vi "storeADCMixedToArray-wang-test2simplifié.vi"(0 "String":string) -> (18 "Graph Data":T1)   [LabVIEW 2014]
uses:
  main/controls/Graph Data.ctl
  <vilib>/Utility/miscctls.llb/LVAnnotationListTypeDef.ctl
  <vilib>/Utility/miscctls.llb/LVCursorListTypeDef.ctl
panel:
  out "Numeric 3":i32
  out "TotalTrigger 2":i32
  out "Array - Numeric":i32[](array[numeric])
  out "counter":i32
  in  "counterc":i32
  out "header string":string
  out "channel":u8[](array[numeric])
  out "Waveform":waveform(dbl)
  out "Graph":waveform(i32)[](graph)
  out "Numeric 2":i32
  out "Numeric":i32
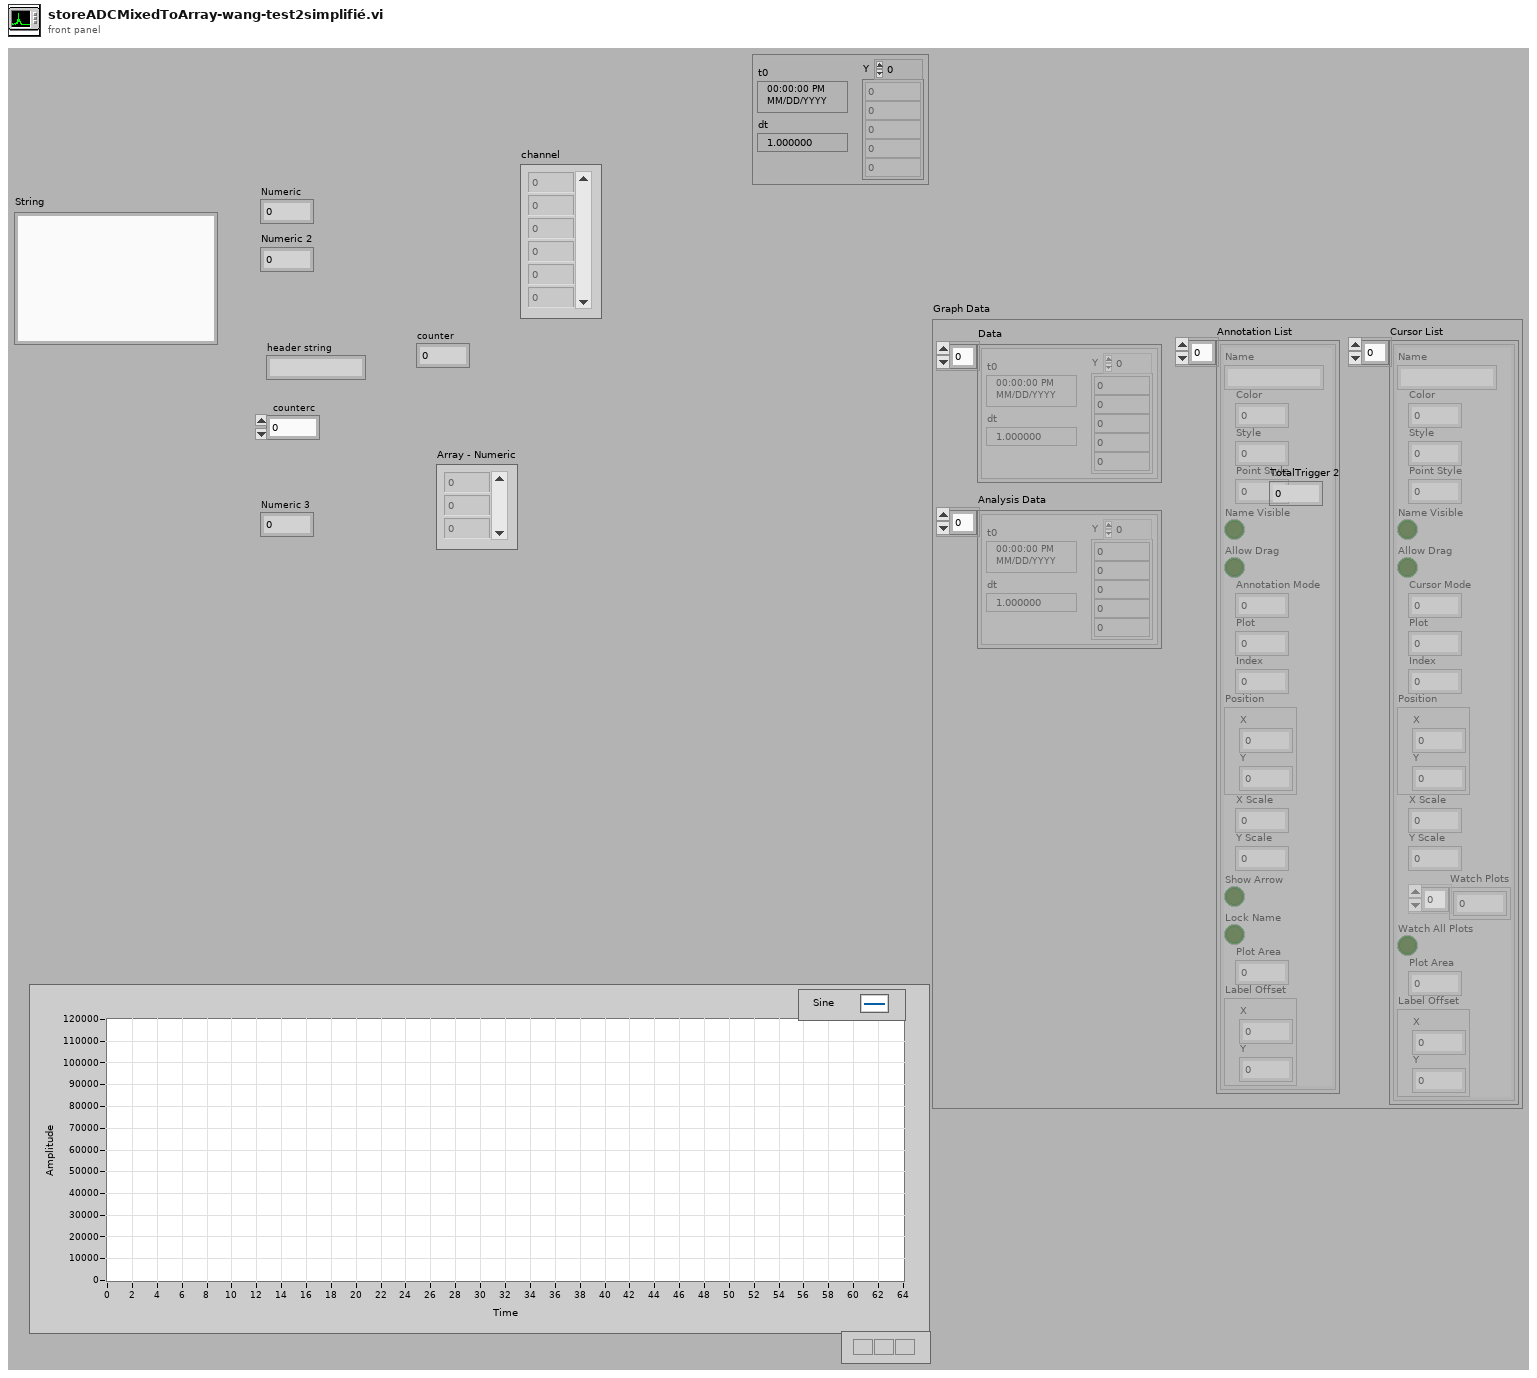
[diagram p1: front panel]
types:
  T1 = typedef "Graph Data.ctl" = cluster{"Data":waveform(dbl)[], "Annotation List":T2, "Cursor List":T3, "Analysis Data":waveform(dbl)[]}
  T2 = typedef "LVAnnotationListTypeDef.ctl" = cluster{"Name":string, "Color":u32, "Style":u8, "Point Style":u8, "Name Visible":bool, "Allow Drag":bool, "Annotation Mode":u32, "Plot":i32, "Index":i32, "Position":cluster{"X":dbl, "Y":dbl}, "X Scale":u32, "Y Scale":u32, "Show Arrow":bool, "Lock Name":bool, "Plot Area":i32, "Label Offset":cluster{"X":dbl, "Y":dbl}}[]
  T3 = typedef "LVCursorListTypeDef.ctl" = cluster{"Name":string, "Color":u32, "Style":u8, "Point Style":u8, "Name Visible":bool, "Allow Drag":bool, "Cursor Mode":u32, "Plot":i32, "Index":i32, "Position":cluster{"X":dbl, "Y":dbl}, "X Scale":u32, "Y Scale":u32, "Watch Plots":i32[], "Watch All Plots":bool, "Plot Area":i32, "Label Offset":cluster{"X":dbl, "Y":dbl}}[]
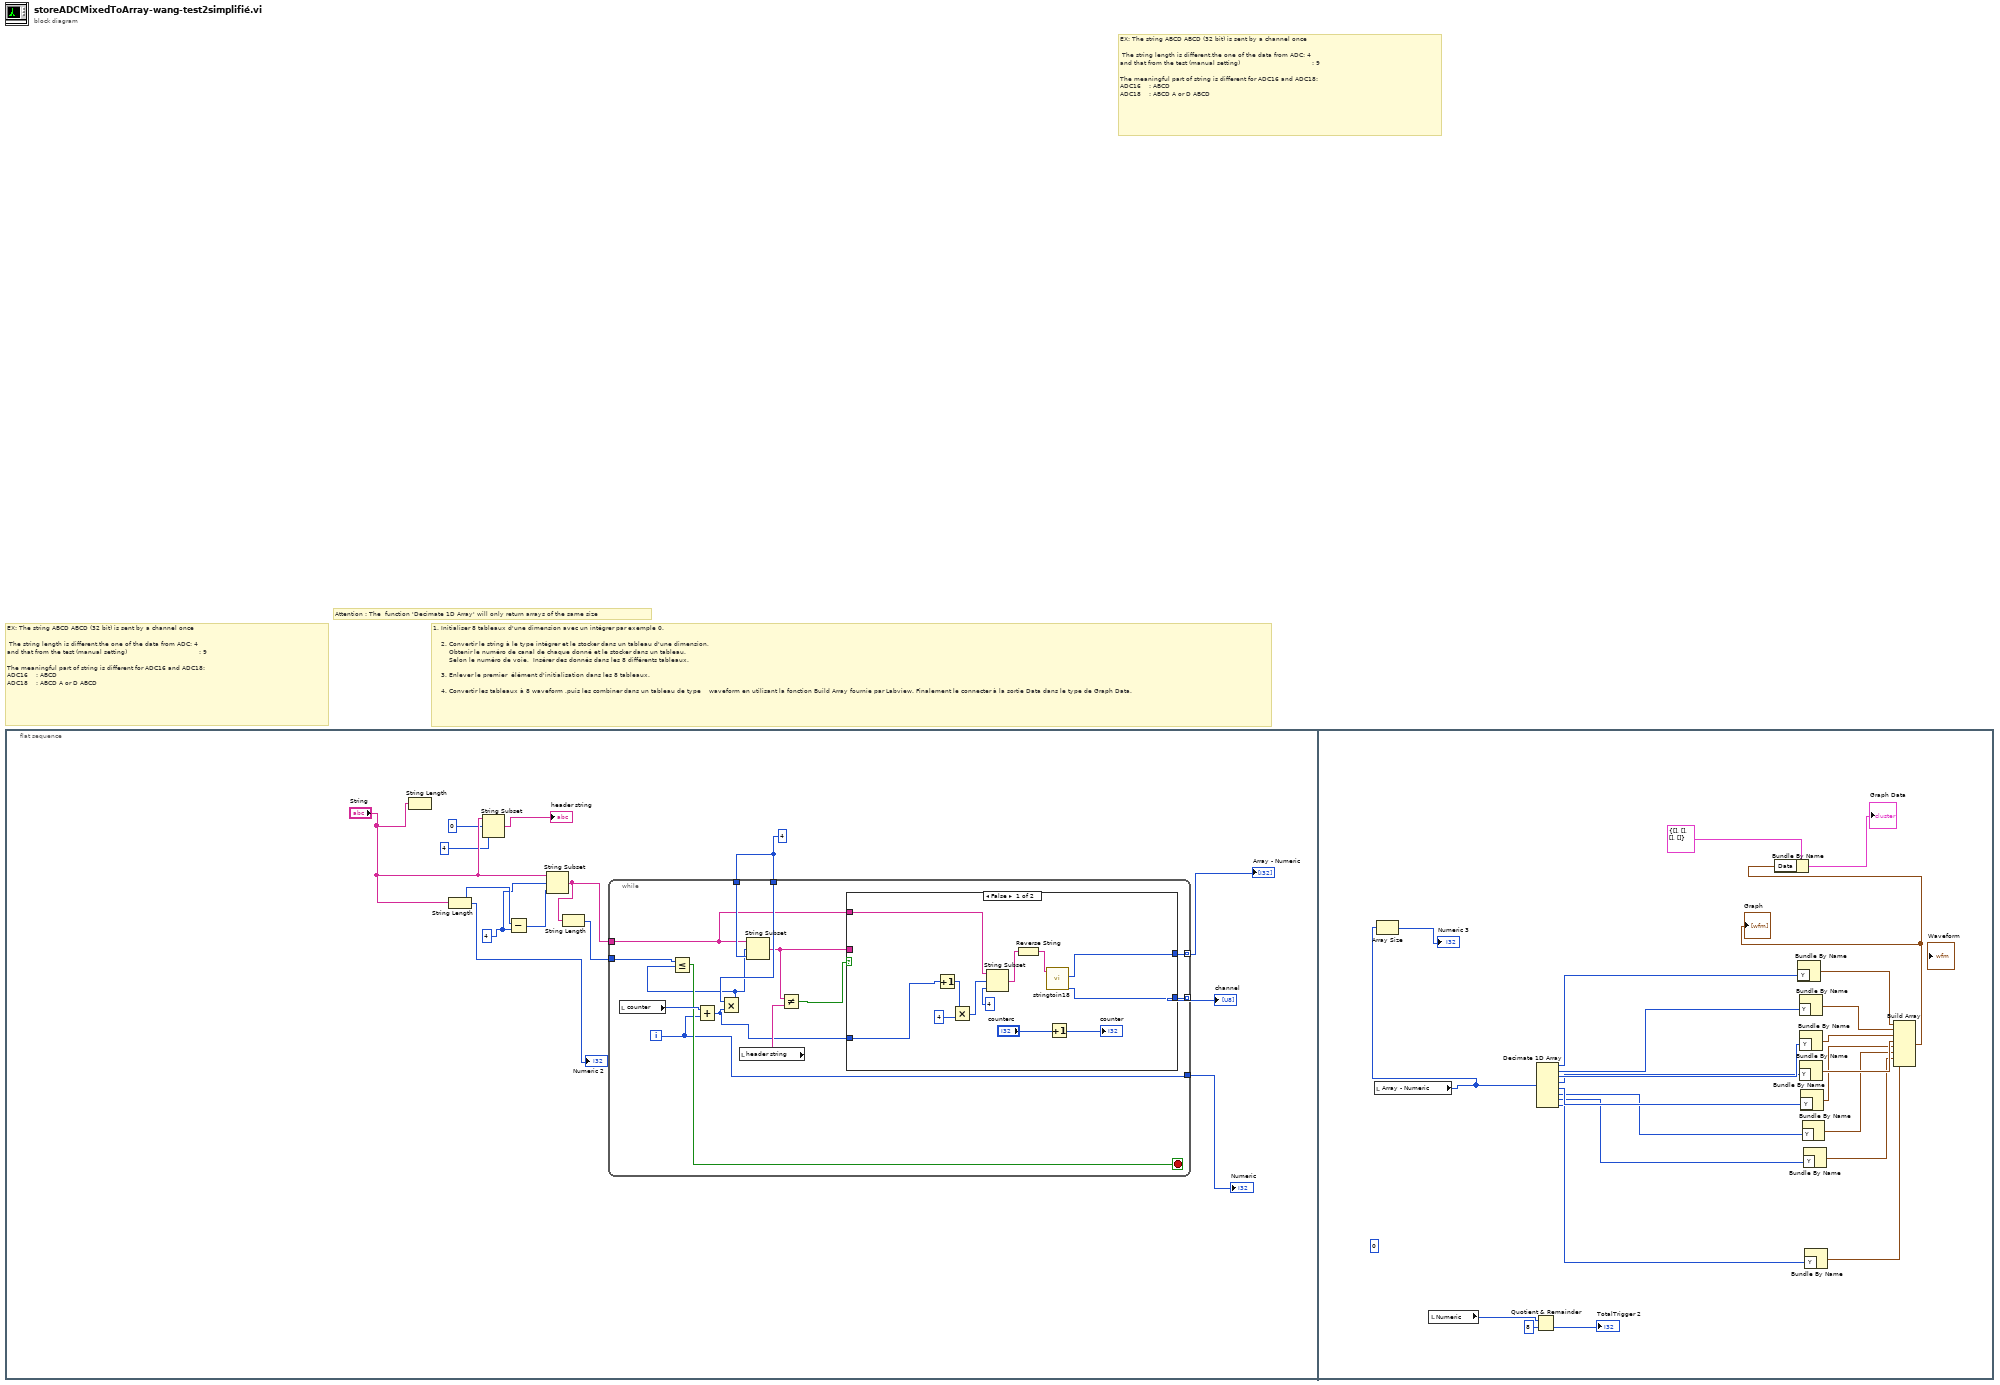
[diagram p0: block diagram]
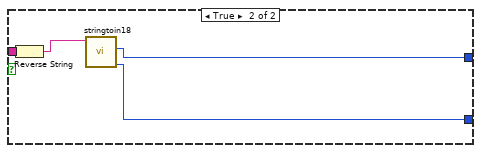
[diagram p2: hidden frame]
diagram:
  # "Attention : The  function 'Decimate 1D Array' will only return arrays of the same size"
  # "1. Initialiser 8 tableaux d'une dimension avec un intégrer par exemple 0.\n\n    2.\tConvertir le string à le type intégrer et le stocker dans un tableau d'une dimension,\n        Obtenir le numéro de canal de chaque donné et le stocker dans un tableau.  \n        Selon le numéro de voie,  Insérer des donnés dans les 8 différents tableaux.\n\n    3. Enlever le premier  élément d'initialisation dans les 8 tableaux.\n\n    4. Convertir les tableaux à 8 waveform ,puis les combiner dans un tableau de type    waveform en utilisant la fonction Build Array fournie par Labview. Finalement le connecter à la sortie Data dans le type de Graph Data."
  # "EX: The string ABCD ABCD (32 bit) is sent by a channel once                \n\n The string length is different,the one of the data from ADC: 4\nand that from the test (manual setting)                                    : 9\n\nThe meaningful part of string is different for ADC16 and ADC18:\nADC16    : ABCD                          \nADC18    : ABCD A or D ABCD"
  # "EX: The string ABCD ABCD (32 bit) is sent by a channel once                \n\n The string length is different,the one of the data from ADC: 4\nand that from the test (manual setting)                                    : 9\n\nThe meaningful part of string is different for ADC16 and ADC18:\nADC16    : ABCD                          \nADC18    : ABCD A or D ABCD"
  n1 = flat-sequence {
    frame #0 {
      w2 = 4
      w5 = 4
      n2 = String Length(string="String") -> ()  [unwired: 1 out]
      n3 = String Length(string="String") -> (length=w13:i32)
      "Numeric 2" <- w13
      n4 = String Subset(string="String", offset (0)=0, length (rest)=4 ("length (rest)")) -> (substring=→"header string":string)
      n5 = Subtract(x=w13, y=w5) -> (x-y=w11:i32)
      n6 = String Subset(string="String", offset (0)=w5, length (rest)=w11) -> (substring=w4:string)
      n7 = String Length(string=w4) -> (length=w3:i32)
      n8 = while {
        tunnel: w2 -> [w27]
        tunnel: w2 -> [w26]
        tunnel: [w16] -> w12
        tunnel: w4 -> [w21]
        tunnel: [w25] -> w1 mode=indexing
        tunnel: [w24] -> w10 mode=indexing
        tunnel: w3 -> [w18]
        i -> [w16]
        stop <- w17 stop-if-true
        n9 = local read "counter"() -> (w22:i32)
        n10 = Add(x=w22, y=w16) -> (x+y=w14:i32)
        n11 = Multiply(x=w26, y=w14) -> (x*y=w15:i32)
        n12 = Less Or Equal?(x=w18, y=w15) -> (x <= y?=w17:bool)
        n13 = local read "header string"() -> (w23:string)
        n14 = String Subset(string=w21, offset (0)=w15, length (rest)=w27) -> (substring=w20:string)
        n15 = Not Equal?(x=w20, y=w23) -> (x != y?=w19:bool)
        n16 = case shown="False" w19 {
          tunnel: [w35 w43] -> w25
          tunnel: [w34 w42] -> w24
          tunnel: w20 -> [_ w40]
          tunnel: w21 -> [w38 _]
          tunnel: w14 -> [w28 _]
          frame False {
            n17 = Increment(x=w28) -> (x+1=w32:i32)
            n18 = Multiply(x=w32, y=4) -> (x*y=w31:i32)
            n19 = String Subset(string=w38, offset (0)=w31, length (rest)=4) -> (substring=w37:string)
            n20 = Reverse String(1:w37) -> (0:w36:string)
            n21 = call "stringtoin18.vi"("input_string"=w36) -> ("channel"=w34:u8, "outputComplemented_int"=w35:i32)  [unwired: 7 in, 2 out]
            n22 = Increment(x="counterc") -> (x+1=→"counter":i32)
          }
          frame True {
            n23 = Reverse String(1:w40) -> (0:w41:string)
            n24 = call "stringtoin18.vi"("input_string"=w41) -> ("channel"=w42:u8, "outputComplemented_int"=w43:i32)  [unwired: 7 in, 2 out]
          }
        }
      }
      "Numeric" <- w12
      "channel" <- w10
      "Array - Numeric" <- w1
    }
    frame #1 {
      (unwired) 0
      n25 = local read "Array - Numeric"() -> (w46:i32[])
      n26 = Array Size(array=w46) -> (size(s)=→"Numeric 3":i32)
      n27 = local read "Numeric"() -> (w45:i32)
      n28 = Quotient & Remainder(x=w45, y=8) -> (floor(x/y)=→"TotalTrigger 2":i32)  [unwired: 1 out]
      n29 = Decimate 1D Array(w46) -> (w56:i32[], w55:i32[], w54:i32[], w53:i32[], w52:i32[], w51:i32[], w50:i32[], w49:i32[])
      n30 = Bundle By Name("Y"=w56) -> (w67:waveform(i32))  [unwired: 1 in]
      n31 = Bundle By Name("Y"=w55) -> (w66:waveform(i32))  [unwired: 1 in]
      n32 = Bundle By Name("Y"=w53) -> (w64:waveform(i32))  [unwired: 1 in]
      n33 = Bundle By Name("Y"=w54) -> (w65:waveform(i32))  [unwired: 1 in]
      n34 = Bundle By Name("Y"=w52) -> (w60:waveform(i32))  [unwired: 1 in]
      n35 = Bundle By Name("Y"=w51) -> (w63:waveform(i32))  [unwired: 1 in]
      n36 = Bundle By Name("Y"=w50) -> (w62:waveform(i32))  [unwired: 1 in]
      n37 = Bundle By Name("Y"=w49) -> (w61:waveform(i32))  [unwired: 1 in]
      n38 = Build Array(w67, w66, w65, w64, w60, w63, w62, w61) -> (w59:waveform(i32)[])
      "Graph" <- w59
      n39 = Bundle By Name(cluster=T1 {"Data"=[], "Annotation List"=[], "Cursor List"=[], "Analysis Data"=[]} ("Graph Data"), "Data"=w59) -> (→"Graph Data":T1)
    }
  }
